vi "DB Update.vi"(6 "Where":string, 7 "table Name":string, 8 "error in (no error)":errorcluster, 9 "Column Name":string[](array[string]), 10 "Column Values":string[](array[string]), 11 "Db Reference":refnum<k24>) -> (0 "error out":errorcluster, 2 "data":i32, 3 "Db Reference":refnum<k24>)   [LabVIEW 2020]
uses:
  D:/Labview/Auto Run Screen/Source Code/Database/Support/dbquery.dll
  Support/dbquery.dll
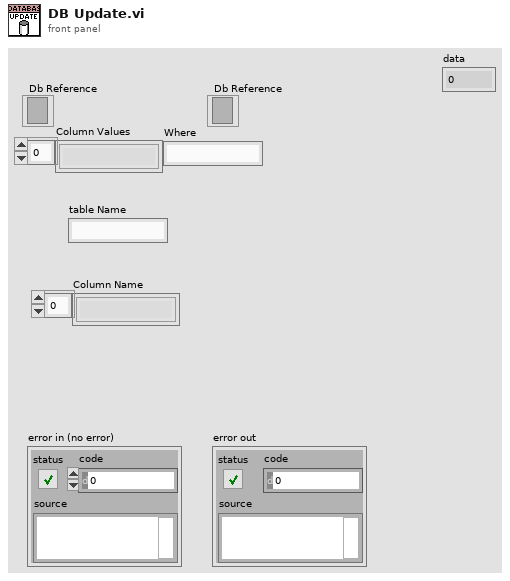
[diagram p1: front panel]
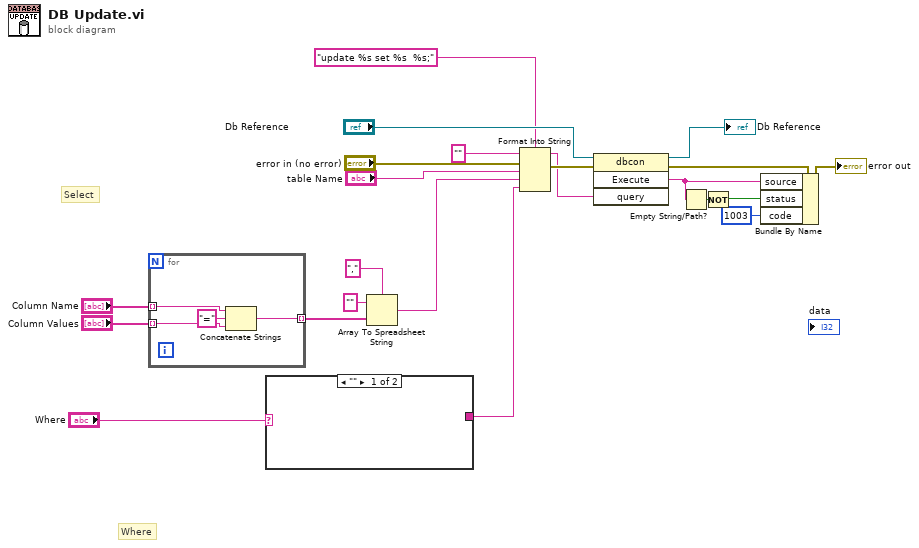
[diagram p0: block diagram]
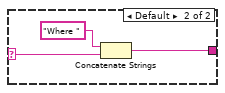
[diagram p2: hidden frame]
diagram:
  # "Where"
  # "Select"
  n1 = for {
    tunnel: "Column Name" -> [w26] mode=indexing
    tunnel: "Column Values" -> [w25] mode=indexing
    tunnel: [w23] -> w10 mode=indexing
    n2 = Concatenate Strings(w26, "=" ("string"), w25) -> (w23:string)
  }
  n3 = case shown="\"\"" "Where" {
    selector: "Where" -> [_ w27]
    tunnel: [_ w29] -> w8
    frame "" {
    }
    frame Default {
      n4 = Concatenate Strings("Where " ("string"), w27) -> (w29:string)
    }
  }
  n5 = Array To Spreadsheet String(delimiter (Tab)=",", array=w10, 3:"" ("format string")) -> (spreadsheet string=w9:string)
  n6 = Format Into String(format string="update %s set %s  %s;", initial string="", error in="error in (no error)", "table Name", w9, w8) -> (resulting string=w15:string, error out=w16:errorcluster)
  n7 = invoke class="dbcon" method="Execute"(reference="Db Reference", error in=w16, "query"=w15) -> (reference out=→"Db Reference":refnum<k24>, error out=w7:errorcluster, "Execute"=w5:string)  [unwired: 1 in, 1 out]
  n8 = Empty String/Path?(string/path=w5) -> (empty?=w4:bool)
  n9 = Not(x=w4) -> (.not. x?=w3:bool)
  n10 = Bundle By Name(cluster=w7, "source"=w5, "status"=w3, "code"=1003) -> (→"error out":errorcluster)
